vi "Refresh MCL.vi"(8 "Error In":errorcluster) -> (0 "Error Out":errorcluster)   [LabVIEW 2023, in "Error Manager.lvlib"]
doc: "Blank VI with error handling."
uses:
  Error Manager.lvlib
  Queues/MHL Queue/Command (enum).ctl
  Queues/MHL Queue/MHL Queue.lvclass
panel:
  # "Input\nInputs to the VI"
  # "Development\nControls or indicators that are useful for development or testing, but which are not outputs of the VI."
  # "Output\nOutputs of the VI"
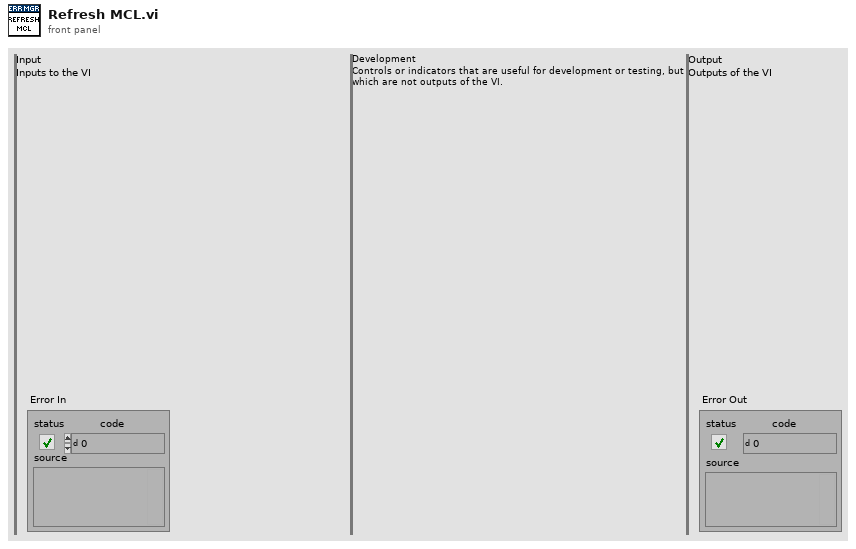
[diagram p1: front panel]
types:
  T1 = typedef "Error Manager.lvlib/MHL Queue.lvclass/Command (enum).ctl" = enum16{"Init Module", "Close Module", "Internal Error", "Create Error Log File", "Show Front Panel", "Handle Error", "Refresh MCL", "MCL Value Change", "Mark Error As Read", "Mark All Errors As Read", "Change Display Order", "One-Second Interval Expired"}
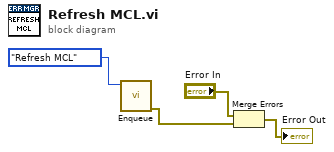
[diagram p0: block diagram]
diagram:
  n1 = call "Enqueue.vi"(11:Command_(enum)."Refresh MCL" ("Command")) -> (0:w3:errorcluster)  [unwired: 10 in]
  n2 = Merge Errors("Error In", w3) -> (→"Error Out":errorcluster)
